vi "Merge Runner.vi"(10 "Test Runner":refnum<class "Test Runner.lvclass">, 11 "Test Runner.Collection in":refnum<class "Test Runner.Collection.lvclass">) -> (3 "Test Runner.Collection out":refnum<class "Test Runner.Collection.lvclass">)   [LabVIEW 2013, in "Caraya.lvlib" / "Test Runner.Collection.lvclass"]
uses:
  Test Runner.Collection.lvclass
  Test Runner/Test Runner.lvclass
  Test Runner.Collection.lvclass/Test Runner.Collection.ctl
  Test Runner/Test Runner.lvclass/Test Runner.ctl
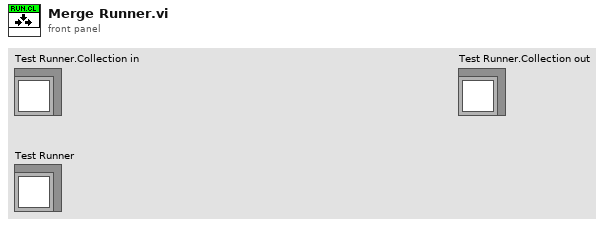
[diagram p1: front panel]
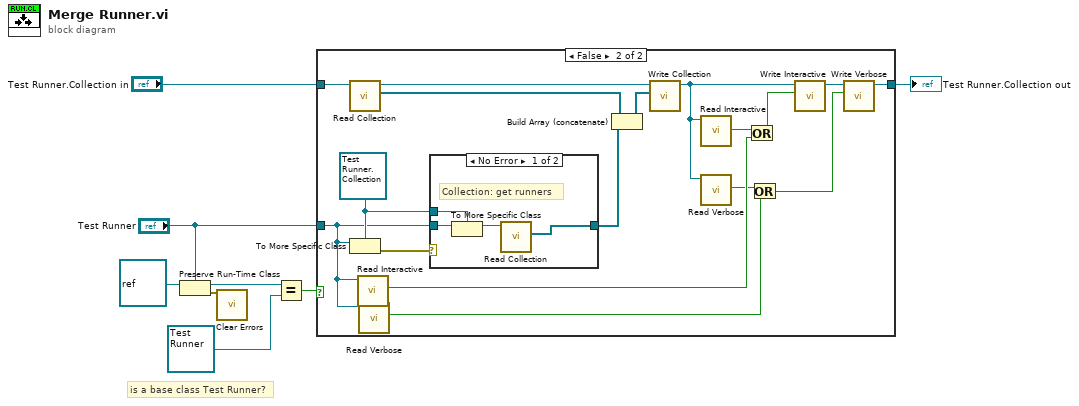
[diagram p0: block diagram]
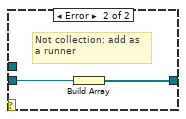
[diagram p3: hidden frame]
diagram:
  # "is a base class Test Runner?"
  n1 = Preserve Run-Time Class(object in=refnum<class> refnum ("LabVIEW Object"), 2:"Test Runner") -> (object out=w4:refnum<class "Test Runner.lvclass">, error out=w1:errorcluster)  [unwired: 1 in]
  n2 = call <vilib>:"Clear Errors.vi"("error in (no error)"=w1) -> ()  [unwired: 6 in, 1 out]
  n3 = Equal?(x=w4, y=refnum<class "Test Runner.lvclass"> refnum ("Caraya.lvlib:Test Runner.lvclass")) -> (x = y?=w2:bool)
  n4 = case shown="False" w2 {
    tunnel: [w9 w13] -> w8
    tunnel: "Test Runner.Collection in" -> [w9 w20]
    tunnel: "Test Runner" -> [_ w19]
    frame True {
    }
    frame False {
      w24 = refnum<class "Test Runner.Collection.lvclass"> refnum ("Collection")
      n5 = call "Read Collection.vi"("Test Runner.Collection in"=w20) -> ("Test Runners"=w22:refnum<class "Test Runner.lvclass">[], "Test Runner.Collection out"=w21:refnum<class "Test Runner.Collection.lvclass">)  [unwired: 9 in]
      n6 = To More Specific Class(target class=w24, reference=w19) -> (error out=w23:errorcluster)  [unwired: 1 in, 1 out]
      n7 = call "Read Interactive.vi"("Test Runner in"=w19) -> ("Interactive"=w15:bool)  [unwired: 9 in, 1 out]
      n8 = call "Read Verbose.vi"("Test Runner in"=w19) -> ("Verbose"=w11:bool)  [unwired: 9 in, 1 out]
      n9 = case shown="No Error" w23 {
        tunnel: w19 -> [w29 w31]
        tunnel: [w30 w32] -> w25
        tunnel: w24 -> [w28 _]
        frame No Error {
          # "Collection: get runners"
          n10 = To More Specific Class(target class=w28, reference=w29) -> (specific class reference=w27:refnum<class "Test Runner.Collection.lvclass">)  [unwired: 1 in, 1 out]
          n11 = call "Read Collection.vi"("Test Runner.Collection in"=w27) -> ("Test Runners"=w30:refnum<class "Test Runner.lvclass">[])  [unwired: 9 in, 1 out]
        }
        frame Error {
          # "Not collection: add as\na runner"
          n12 = Build Array(w31) -> (w32:refnum<class "Test Runner.lvclass">[])
        }
      }
      n13 = Build Array (concatenate)(w22, w25) -> (w26:refnum<class "Test Runner.lvclass">[])
      n14 = call "Write Collection.vi"("Collection"=w26, "Test Runner.Collection in"=w21) -> ("Test Runner.Collection out"=w17:refnum<class "Test Runner.Collection.lvclass">)  [unwired: 8 in, 1 out]
      n15 = call "Read Interactive.vi"("Test Runner in"=w17) -> ("Interactive"=w18:bool)  [unwired: 9 in, 1 out]
      n16 = call "Read Verbose.vi"("Test Runner in"=w17) -> ("Verbose"=w12:bool)  [unwired: 9 in, 1 out]
      n17 = Or(x=w18, y=w15) -> (x .or. y?=w16:bool)
      n18 = Or(x=w12, y=w11) -> (x .or. y?=w10:bool)
      n19 = call "Write Interactive.vi"("Interactive"=w16, "Test Runner in"=w17) -> ("Test Runner out"=w14:refnum<class "Test Runner.Collection.lvclass">)  [unwired: 9 in]
      n20 = call "Write Verbose.vi"("Verbose"=w10, "Test Runner in"=w14) -> ("Test Runner out"=w13:refnum<class "Test Runner.Collection.lvclass">)  [unwired: 9 in]
    }
  }
  "Test Runner.Collection out" <- w8
